vi "loop_data_conversion_factor.vi"(1 "from analog?":bool=TRUE) -> (0 "MATLAB function handler":string[](array[string]))   [LabVIEW 2017]
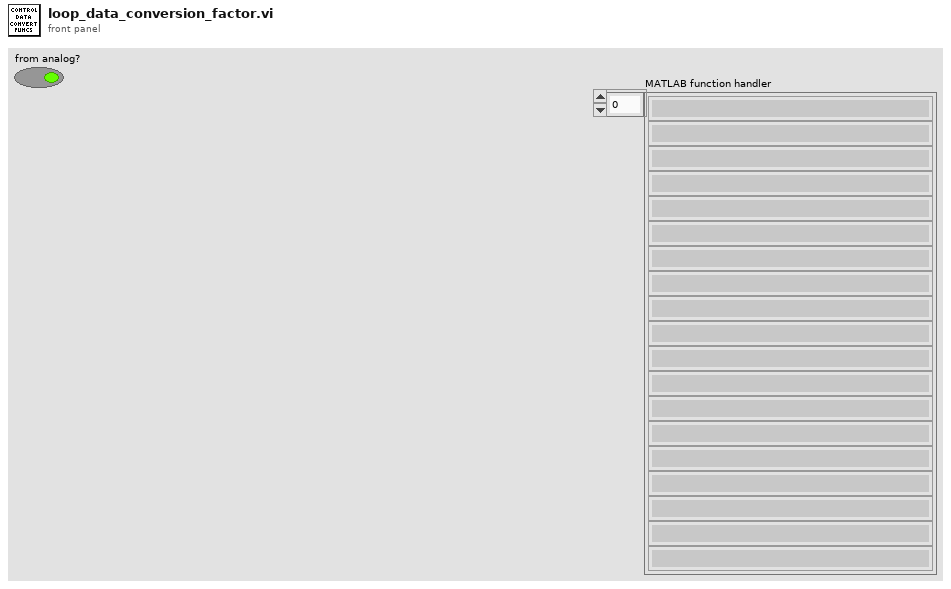
[diagram p1: front panel]
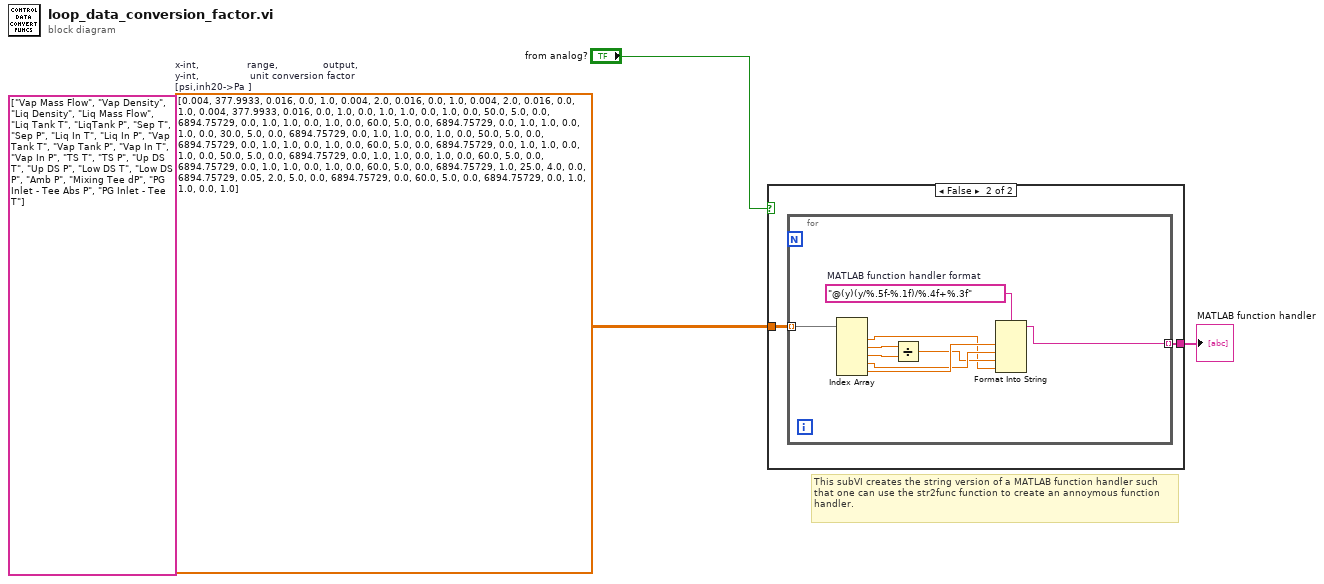
[diagram p0: block diagram]
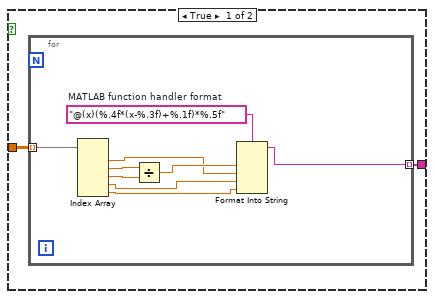
[diagram p2: hidden frame]
diagram:
  w3 = dbl[][] [[0.004, 377.9933, 0.016, 0.0, 1.0], [0.004, 2.0, 0.016, 0.0, 1.0], [0.004, 2.0, 0.016, 0.0, 1.0], [0.004, 377.9933, 0.016, 0.0, 1.0], [0.0, 1.0, 1.0, 0.0, 1.0], [0.0, 50.0, 5.0, 0.0, 6894.75729], [0.0, 1.0, 1.0, 0.0, 1.0], [0.0, 60.0, 5.0, 0.0, 6894.75729], [0.0, 1.0, 1.0, 0.0, 1.0], [0.0, 30.0, 5.0, 0.0, 6894.75729], [0.0, 1.0, 1.0, 0.0, 1.0], [0.0, 50.0, 5.0, 0.0, 6894.75729], [0.0, 1.0, 1.0, 0.0, 1.0], [0.0, 60.0, 5.0, 0.0, 6894.75729], [0.0, 1.0, 1.0, 0.0, 1.0], [0.0, 50.0, 5.0, 0.0, 6894.75729], [0.0, 1.0, 1.0, 0.0, 1.0], [0.0, 60.0, 5.0, 0.0, 6894.75729], [0.0, 1.0, 1.0, 0.0, 1.0], [0.0, 60.0, 5.0, 0.0, 6894.75729], [1.0, 25.0, 4.0, 0.0, 6894.75729], [0.05, 2.0, 5.0, 0.0, 6894.75729], [0.0, 60.0, 5.0, 0.0, 6894.75729], [0.0, 1.0, 1.0, 0.0, 1.0]]  # x-int,                range,               output,           y-int,                 unit conversion factor [psi,inh20->Pa ]
  (unwired) string[] ["Vap Mass Flow", "Vap Density", "Liq Density", "Liq Mass Flow", "Liq Tank T", "LiqTank P", "Sep T", "Sep P", "Liq In T", "Liq In P", "Vap Tank T", "Vap Tank P", "Vap In T", "Vap In P", "TS T", "TS P", "Up DS T", "Up DS P", "Low DS T", "Low DS P", "Amb P", "Mixing Tee dP", "PG Inlet - Tee Abs P", "PG Inlet - Tee T"] ("subarray")
  # "This subVI creates the string version of a MATLAB function handler such that one can use the str2func function to create an annoymous function handler."
  n1 = case shown="False" "from analog?" {
    tunnel: w3 -> [w5 w16]
    tunnel: [w4 w15] -> w2
    frame True {
      n2 = for {
        tunnel: w5 -> [w14] mode=indexing
        tunnel: [w6] -> w4 mode=indexing
        w9 = "@(x)(%.4f*(x-%.3f)+%.1f)*%.5f"  # MATLAB function handler format
        n3 = Index Array(array=w14) -> (element #1=w7:dbl, element #2=w13:dbl, element #3=w12:dbl, element #4=w11:dbl, element #5=w10:dbl)  [unwired: 5 in]
        n4 = Divide(x=w13, y=w12) -> (x/y=w8:dbl)
        n5 = Format Into String(format string=w9, w8, w7, w11, w10) -> (resulting string=w6:string)  [unwired: 2 in, 1 out]
      }
    }
    frame False {
      n6 = for {
        tunnel: w16 -> [w25] mode=indexing
        tunnel: [w21] -> w15 mode=indexing
        w22 = "@(y)(y/%.5f-%.1f)/%.4f+%.3f"  # MATLAB function handler format
        n7 = Index Array(array=w25) -> (element #1=w17:dbl, element #2=w24:dbl, element #3=w23:dbl, element #4=w19:dbl, element #5=w20:dbl)  [unwired: 5 in]
        n8 = Divide(x=w24, y=w23) -> (x/y=w18:dbl)
        n9 = Format Into String(format string=w22, w20, w19, w18, w17) -> (resulting string=w21:string)  [unwired: 2 in, 1 out]
      }
    }
  }
  "MATLAB function handler" <- w2
